vi "Unit Test Engine Global.vi"() -> ()   [LabVIEW 2019, in "Assert.lvlib"]
uses:
  Assert/Assert.lvlib
panel:
  in  "Station(Test Engine)":i32
  in  "Number of Tests Sockets":u8=1 min=1 max=4
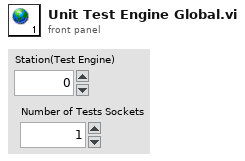
[diagram p1: front panel]
diagram:
